vi "Run.vi"(8 "error in (no error)":errorcluster caption="entrée d'erreur (pas d'erreur)", 9 "Y":string[][](array[string]), 10 "X":string[][](array[string]), 11 "Additive_chi2_kernel.lvclass":refnum<class "Additive_chi2_kernel.lvclass">) -> (0 "error out":errorcluster caption="sortie d'erreur", 2 "Data":T1, 3 "Additive_chi2_kernel.lvclass":refnum<class "Additive_chi2_kernel.lvclass">)   [LabVIEW 2020, in "Additive_chi2_kernel.lvclass"]
doc: "Returns : \n\n- kernel_matrix : array of shape (n_samples_X, n_samples_Y)"
uses:
  Additive_chi2_kernel.lvclass
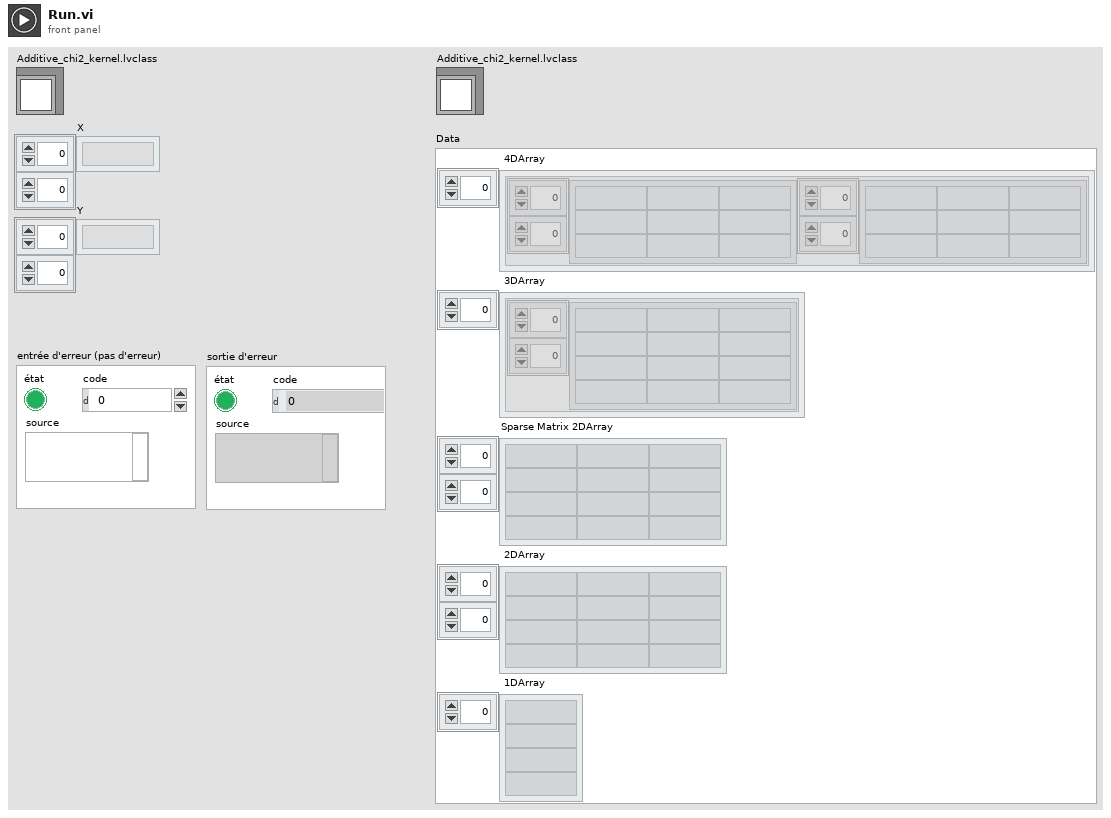
[diagram p1: front panel]
types:
  T1 = cluster{" 4DArray":cluster{"1":string[][], "2":string[][]}[], " 3DArray":cluster{"Tableau":string[][]}[], "Sparse Matrix 2DArray":string[][], " 2DArray":string[][], " 1DArray":string[]}
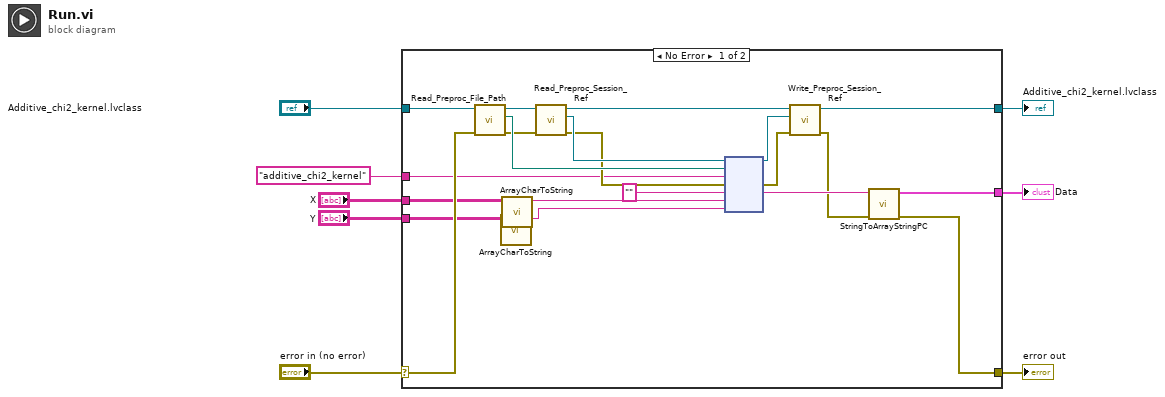
[diagram p0: block diagram]
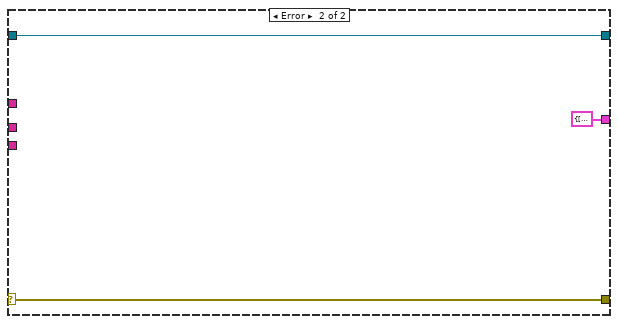
[diagram p2: hidden frame]
diagram:
  n1 = case shown="No Error" "error in (no error)" {
    selector: "error in (no error)" -> [w19 w32]
    tunnel: [w10 w32] -> w7
    tunnel: [w15 w31] -> w5
    tunnel: "Additive_chi2_kernel.lvclass" -> [w20 w31]
    tunnel: "additive_chi2_kernel" ("Fonction") -> [w18 _]
    tunnel: "X" -> [w14 _]
    tunnel: "Y" -> [w13 _]
    tunnel: [w9 T1 {" 4DArray"=[], " 3DArray"=[], "Sparse Matrix 2DArray"=[], " 2DArray"=[], " 1DArray"=[]} ("Data")] -> w1
    frame No Error {
      n2 = call-dynamic "Read_Preproc_File_Path.vi"("error in (no error)"=w19, "Python in"=w20) -> ("error out"=w24:errorcluster, "File_Path"=w27:path, "Python out"=w29:refnum<class "Additive_chi2_kernel.lvclass">)  [unwired: 7 in]
      n3 = call "ArrayCharToString.vi"("TAB"=w13) -> ("Instruction"=w16:string)  [unwired: 10 in]
      n4 = call "ArrayCharToString.vi"("TAB"=w14) -> ("Instruction"=w17:string)  [unwired: 10 in]
      n5 = call-dynamic "Read_Preproc_Session_Ref.vi"("error in (no error)"=w24, "Python in"=w29) -> ("error out"=w25:errorcluster, "Session_ref"=w26:refnum<k35>, "Python out"=w28:refnum<class "Additive_chi2_kernel.lvclass">)  [unwired: 7 in]
      n6 = node(w26, w27, w18, w25, "", w17, w16) -> (w21:refnum<k35>, w23:errorcluster, w12:string)  [unwired: 2 in, 2 out]
      n7 = call-dynamic "Write_Preproc_Session_Ref.vi"("error in (no error)"=w23, "Session_ref"=w21, "Python in"=w28) -> ("error out"=w11:errorcluster, "Python out"=w15:refnum<class "Additive_chi2_kernel.lvclass">)  [unwired: 7 in]
      n8 = call "StringToArrayStringPC.vi"("sortie d'erreur"=w11, "Return value"=w12) -> ("sortie d'erreur"=w10:errorcluster, "Data"=w9:T1)  [unwired: 8 in]
    }
    frame Error {
    }
  }
  "error out" <- w7
  "Additive_chi2_kernel.lvclass" <- w5
  "Data" <- w1
